vi "ResetCredit.vi"(8 "error in (no error)":errorcluster, 11 "Messages Actor in":refnum<class "Messages Actor.lvclass">) -> (0 "error out":errorcluster, 3 "Messages Actor out":refnum<class "Messages Actor.lvclass">)   [LabVIEW 2020, in "Messages Actor.lvlib" / "Messages Actor.lvclass"]
uses:
  Messages Actor.lvclass
  Messages Actor.lvclass/Messages Actor.ctl
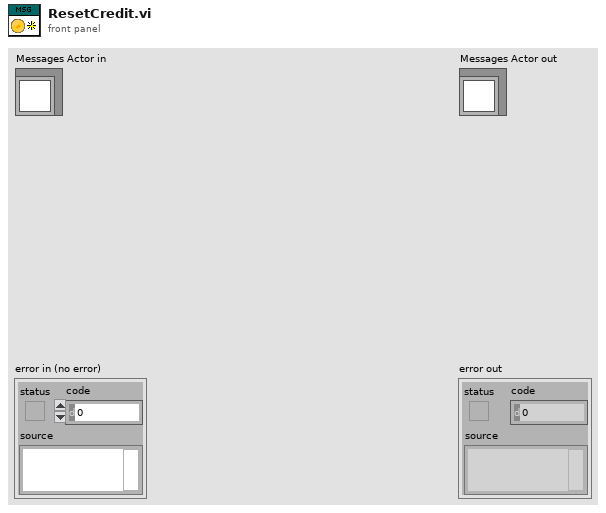
[diagram p1: front panel]
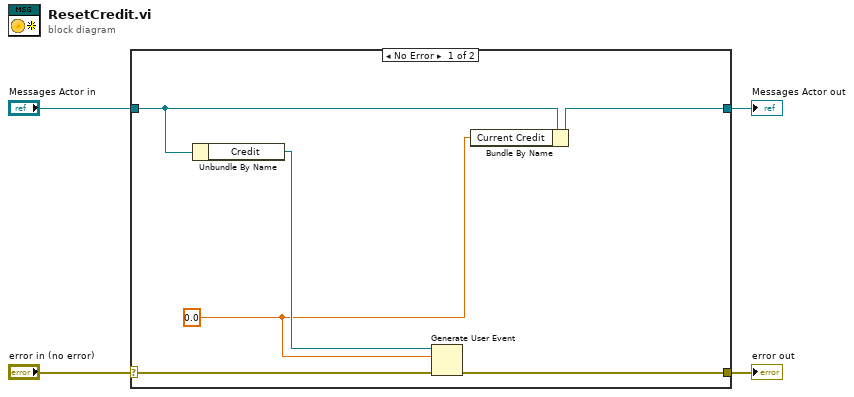
[diagram p0: block diagram]
diagram:
  n1 = case shown="No Error" "error in (no error)" {
    selector: "error in (no error)" -> [w9 w12]
    tunnel: [w8 w12] -> w3
    tunnel: [w10 w11] -> w1
    tunnel: "Messages Actor in" -> [w7 w11]
    frame No Error {
      w5 = 0.0
      n2 = Unbundle By Name(w7) -> ("Credit"=w6:refnum<user-event>)
      n3 = Generate User Event(user event=w6, event data cluster=w5, error in=w9) -> (error out=w8:errorcluster)  [unwired: 1 in, 1 out]
      n4 = Bundle By Name(cluster=w7, "Current Credit"=w5) -> (w10:refnum<class "Messages Actor.lvclass">)
    }
    frame Error {
    }
  }
  "error out" <- w3
  "Messages Actor out" <- w1
